vi "Mindsensors PSPNX Config.vi"(10 "Node Data":T1, 11 "NXT":T2) -> ()   [LabVIEW 2010]
uses:
  <vilib>/NXT/Subs/LVHSConnector.ctl
  Datatypes/Node.ctl
  UI Controls/PlugInControls/Pluginbackground.ctl
  <vilib>/Utility/miscctls.llb/LVPointTypeDef.ctl
  <vilib>/NXT/Block Support/HWPage.SensorMode.ctl
  <vilib>/NXT/Block Support/HWPage.SensorType.ctl
  ConvertNodeAddrSensor.vi
panel:
  out "NXT Port":i16
  out "Right Y":dbl
  out "Right X":dbl
  out "Left Y":dbl
  out "Left X":dbl
  in  "Device Address":string
  in  "Device\n Address":u8=2 format="%x"
  in  "Sensor Parameters":string
  out "number":i8
  out "R 3":bool
  out "L 3":bool
  out "R 2":bool
  out "L 1":bool
  out "R 1":bool
  out "L 2":bool
  out "Start":bool
  out "Select":bool
  out "R":bool
  out "U":bool
  out "L":bool
  out "D":bool
  out "[]":bool
  out "O":bool
  out "^":bool
  out "X":bool
  in  "Name":string
  out "Headline":string="Type (auto populated)"
  in  "Instance Specific Data":cluster{"Example Data":dbl}
  in  "Reset":bool
  in  "Save":bool
  in  "Stop":bool
  out "Background":T3=TRUE
  # "<- No controls below this line"
  # "Common controls such as Buttons, Rings, Sliders, Graphs, Decorations, etc can be found in the <labview>\\Targets\\NI\\NXT\\NXT Toolkit\\Schematic Editor\\UI Controls\\Plugin Controls\\ folder. Use these controls when possible to ensure a consistent look and feel with LabVIEW Education Edition."
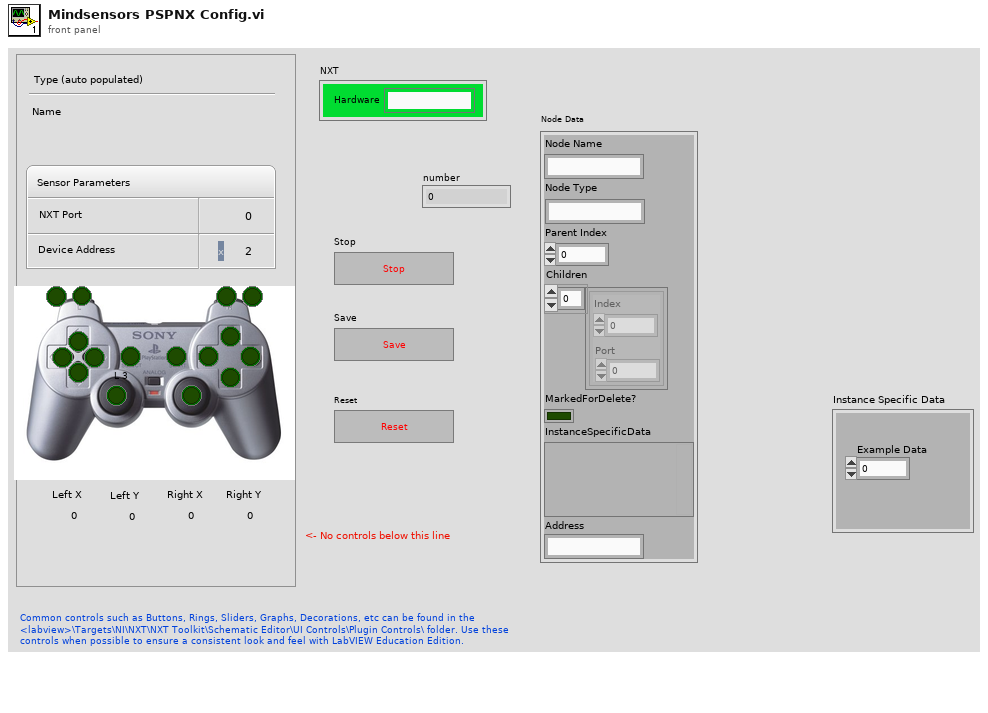
[diagram p1: front panel]
types:
  T1 = typedef "Node.ctl" = cluster{"Node Name":string, "Node Type":string, "Parent Index":i16, "Children":cluster{"Index":u16, "Port":u16}[], "MarkedForDelete?":bool, "InstanceSpecificData":variant, "Address":string}
  T2 = typedef "LVHSConnector.ctl" = cluster{"Hardware":string, "Flattened String":string}
  T3 = typedef "Pluginbackground.ctl" = bool
  T4 = typedef "LVPointTypeDef.ctl" = cluster{"Horizontal":i16, "Vertical":i16}
  T5 = enum8{"Enabled", "Disabled", "Disabled and Grayed Out"}
  T6 = typedef "HWPage.SensorMode.ctl" = u8
  T7 = typedef "HWPage.SensorType.ctl" = u8
  T8 = typedef "NXT_InputPort.ctl" = u8
  T9 = typedef "nxt.ctl" = cluster{"nxtHandle":u32, "fileHandle":u32, "fileIterHandle":u32, "moduleHandle":u32, "modIterHandle":u32, "nxtIterHandle":u32}
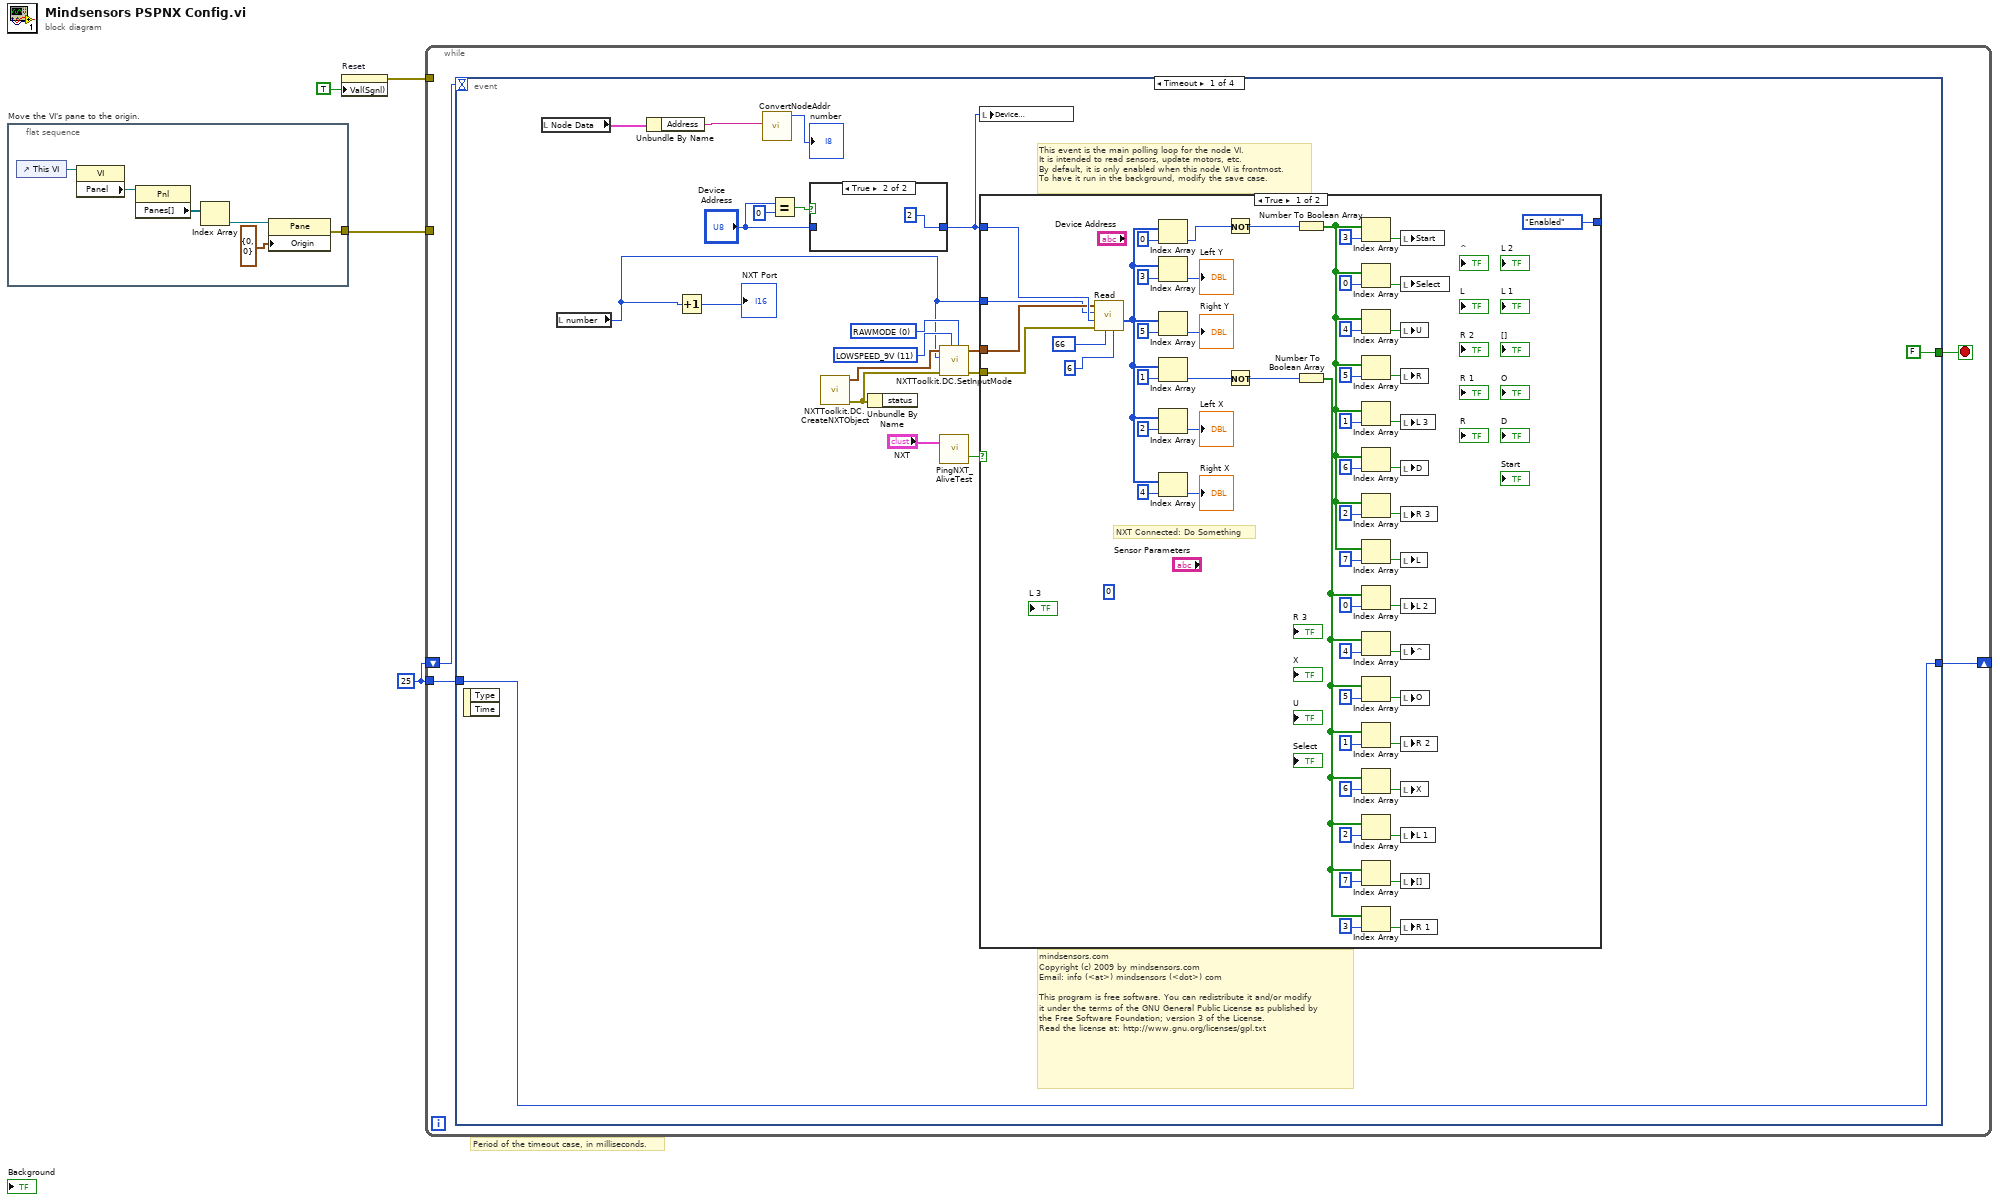
[diagram p0: block diagram]
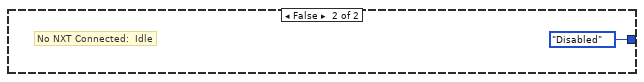
[diagram p3: hidden frame]
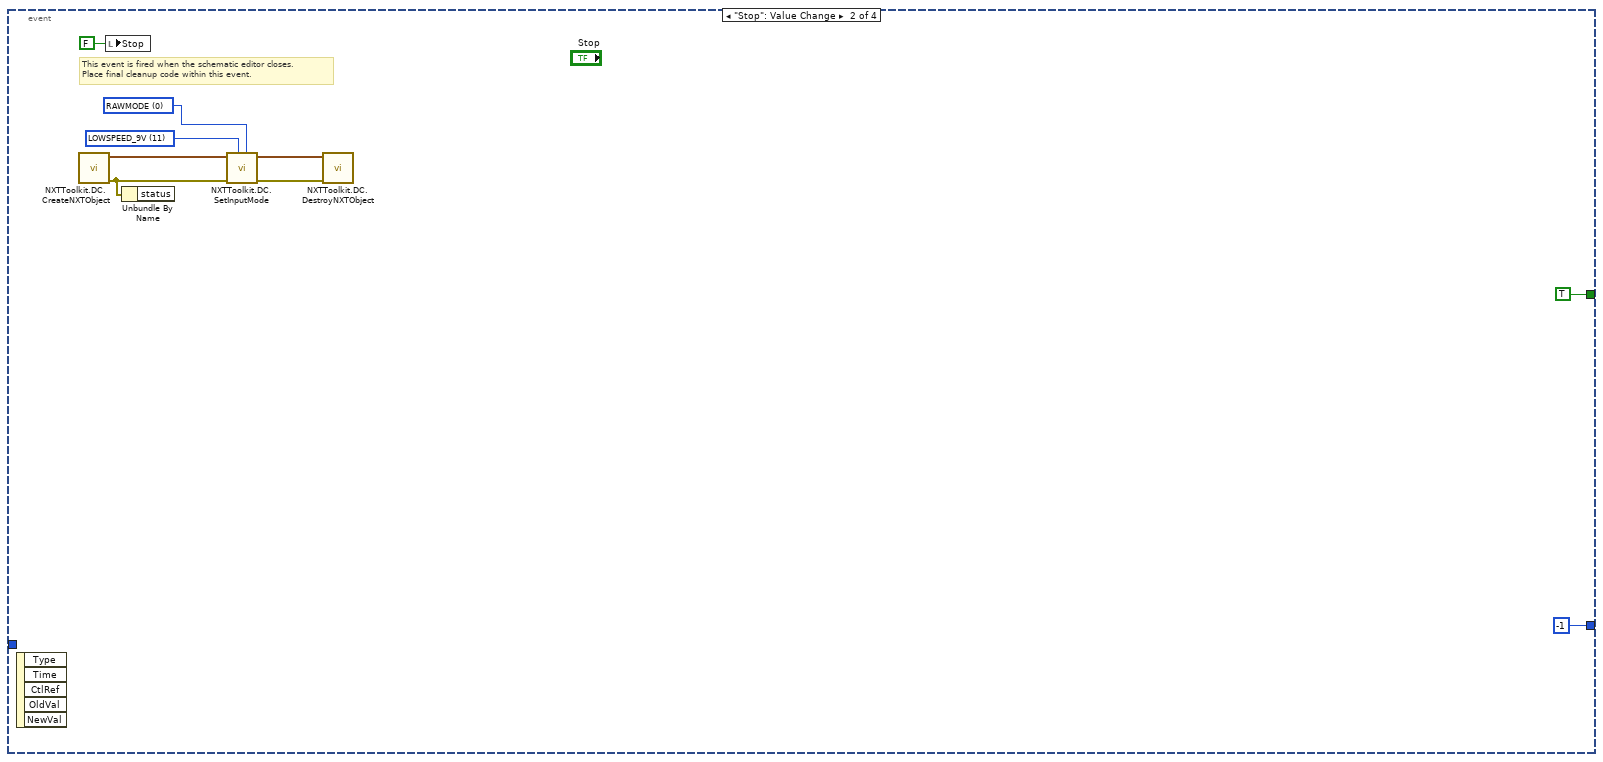
[diagram p4: hidden frame]
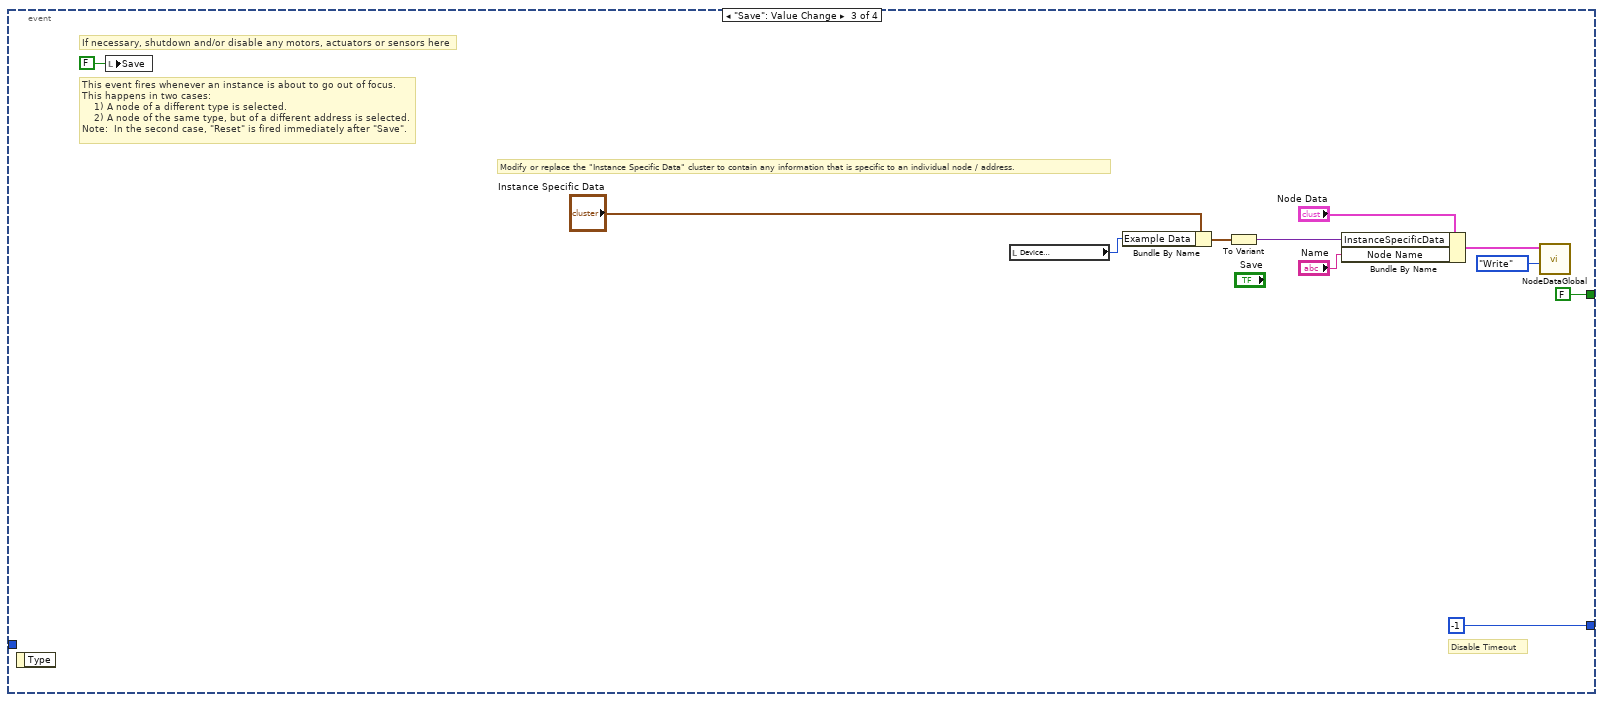
[diagram p5: hidden frame]
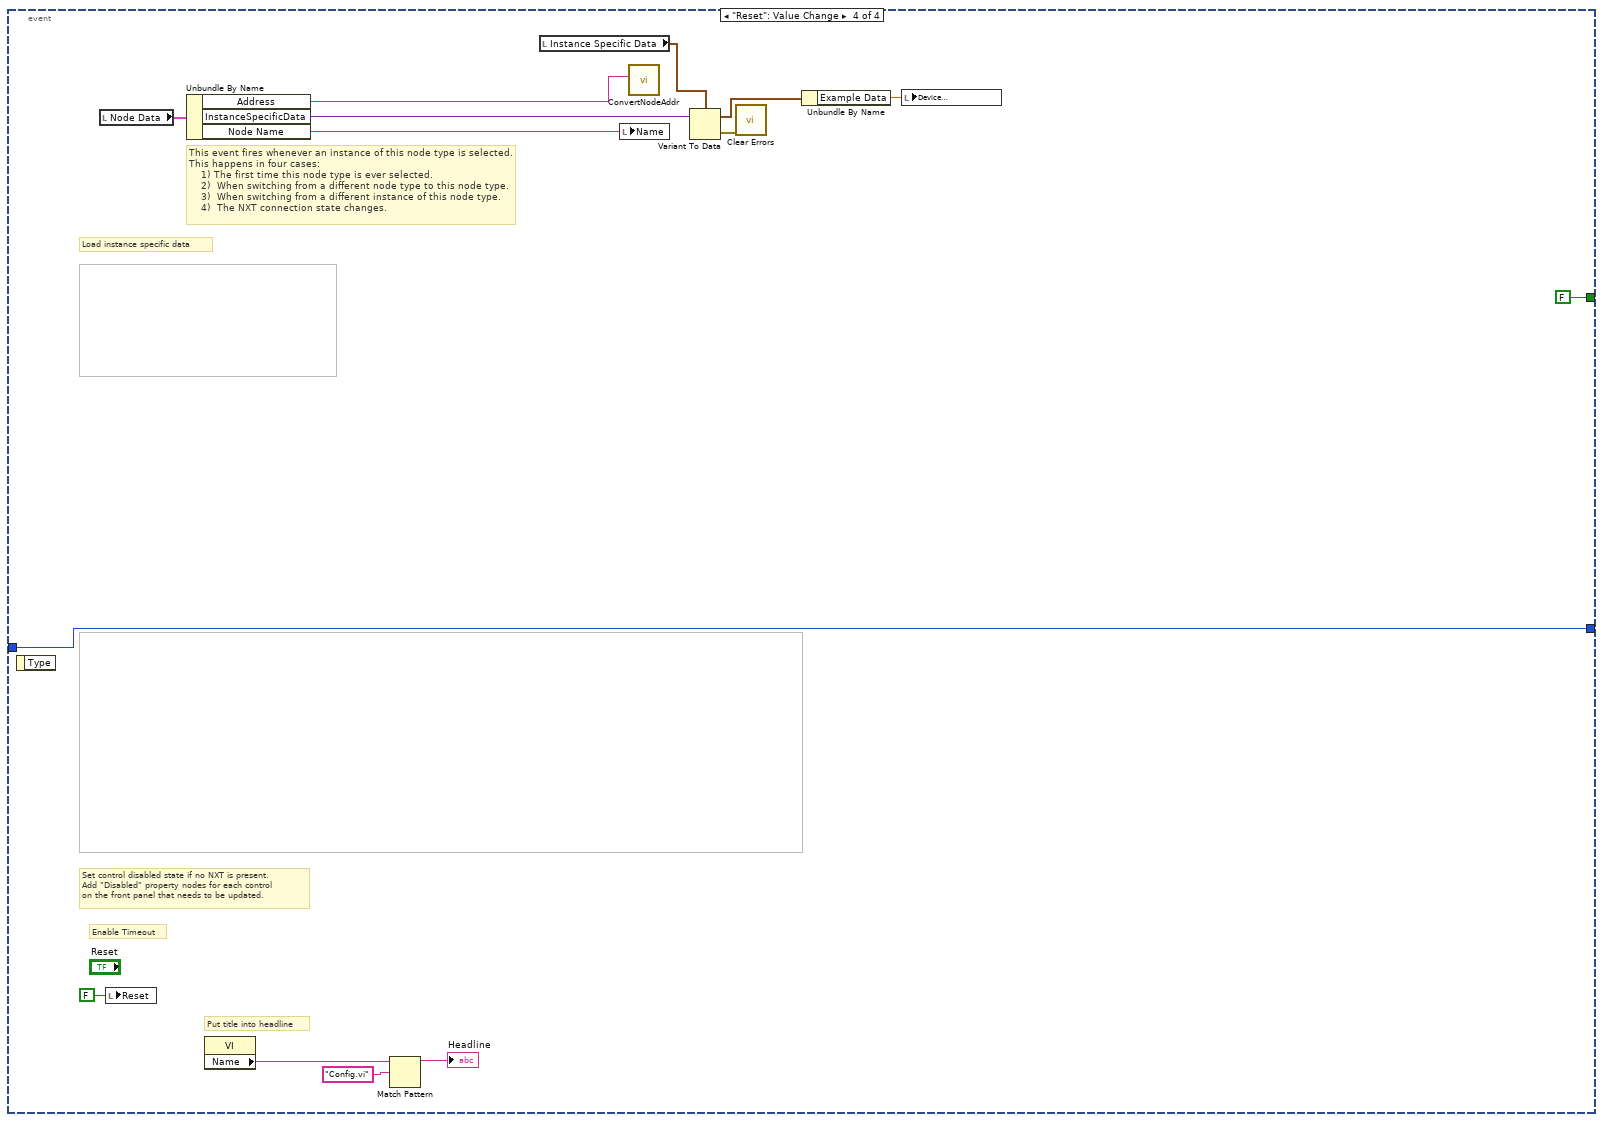
[diagram p6: hidden frame]
diagram:
  w3 = 25
  # "Period of the timeout case, in milliseconds."
  n1 = flat-sequence "Move the VI's pane to the origin." {
    tunnel: [w5] -> w2
    frame #0 {
      n2 = control-ref of="This VI"() -> (w6:refnum<vi>)
      n3 = property class="VI"(reference=w6) -> ("Panel"=w7:refnum<vi>)  [unwired: 1 in, 2 out]
      n4 = property class="Pnl"(reference=w7) -> ("Panes[]"=w8:refnum<vi>[])  [unwired: 1 in, 2 out]
      n5 = Index Array(array=w8) -> (element=w9:refnum<vi>)  [unwired: 1 in]
      n6 = property class="Pane"(reference=w9, "Origin"=T4 {"Horizontal"=0, "Vertical"=0}) -> (error out=w5:errorcluster)  [unwired: 1 in, 1 out]
    }
  }
  n7 = property on="Reset" class="Bool (strict)"("Val(Sgnl)"=TRUE ("Value (Signaling)")) -> (error out=w4:errorcluster)  [unwired: 2 in, 1 out]
  n8 = while {
    tunnel: w4 -> [_]
    shift-right: [w12] -> _
    shift-left: w3 -> [w13]
    tunnel: w3 -> [w11]
    tunnel: w2 -> [_]
    stop <- w14 stop-if-true
    n9 = event shown="[0] Timeout" {
      selector: _ -> [_ _ _ _]
      dyn-events: _ -> [_ _ _ _]
      timeout: w13 -> [_ _ _ _]
      tunnel: [FALSE TRUE FALSE FALSE] -> w14
      tunnel: [w32 -1 -1 w122] -> w12
      tunnel: w11 -> [w32 _ _ w122]
      event Timeout {
        w28 = T6 0 items=["RAWMODE"=0, "BOOLEANMODE"=32, "TRANSITIONCNTMODE"=64, "PERIODCOUNTERMODE"=96, "PCTFULLSCALEMODE"=128, "CELSIUSMODE"=160, "FAHRENHEITMODE"=192, "ANGLESTEPMODE"=224] ("Sensor Mode (RAWMODE)")
        w27 = T7 11 items=["NO_SENSOR", "SWITCH", "TEMPERATURE", "REFLECTION", "ANGLE", "LIGHT_ACTIVE", "LIGHT_INACTIVE", "SOUND_DB", "SOUND_DBA", "CUSTOM", "LOWSPEED", "LOWSPEED_9V", "HIGHSPEED"] ("Sensor Type (NO_SENSOR)")
        # "mindsensors.com\nCopyright (c) 2009 by mindsensors.com\nEmail: info (<at>) mindsensors (<dot>) com\n\nThis program is free software. You can redistribute it and/or modify\nit under the terms of the GNU General Public License as published by\nthe Free Software Foundation; version 3 of the License.\nRead the license at: http://www.gnu.org/licenses/gpl.txt"
        # "This event is the main polling loop for the node VI.\nIt is intended to read sensors, update motors, etc.\nBy default, it is only enabled when this node VI is frontmost.\nTo have it run in the background, modify the save case."
        n10 = event-data() -> ()  [unwired: 1 in, 2 out]
        n11 = local read "Node Data"() -> (w30:T1)
        n12 = local read "number"() -> (w16:i8)
        n13 = Unbundle By Name(w30) -> ("Address"=w18:string)
        n14 = Increment(x=w16) -> (x+1=→"NXT Port":i8)
        n15 = call-poly "ConvertNodeAddr.vi"("Sensor Port"=w18) -> ("NXT Port"=→"number":T8)  [unwired: 6 in, 4 out]
        n16 = Equal?(x="Device\n Address", y=u8 0) -> (x = y?=w21:bool)
        n17 = case shown="True" w21 {
          tunnel: [w34 u8 2 ("Device Addr 2")] -> w19
          tunnel: "Device\n Address" -> [w34 _]
          frame False {
          }
          frame True {
          }
        }
        n18 = call <vilib>:"NXTToolkit.DC.CreateNXTObject.vi"() -> ("error out"=w25:errorcluster, "NXTObject"=w26:T9)  [unwired: 9 in, 1 out]
        n19 = Unbundle By Name(w25) -> ()  [unwired: 1 out]
        n20 = call <vilib>:"NXTToolkit.DC.SetInputMode.vi"("Sensor Mode (RAWMODE)"=w28, "Sensor Type (NO_SENSOR)"=w27, "error in (no error)"=w25, "Input Port (Port 1)"=w16, "NXTObject"=w26) -> ("error out"=w23:errorcluster, "NXTObject dup"=w24:T9)  [unwired: 4 in, 1 out]
        n21 = call <vilib>:"PingNXT_AliveTest.vi"("NXT"="NXT") -> ("connected?"=w29:bool)  [unwired: 1 in, 1 out]
        n22 = local write "Device\n Address"(w19) -> ()
        n23 = case shown="True" w29 {
          tunnel: [T5."Enabled" ("Disabled") T5."Disabled" ("Disabled")] -> _
          tunnel: w16 -> [w36 _]
          tunnel: w19 -> [w90 _]
          tunnel: w24 -> [w38 _]
          tunnel: w23 -> [w37 _]
          frame True {
            (unwired) 0 ("index")
            # "NXT Connected: Do Something"
            n24 = call <vilib>:"Read.vi"("bytes to read"=u8 6, "Reg Address"=u8 66, "error in (no error)"=w37, "Device Address"=w90, "Input Port in"=w36, "NXTObject"=w38) -> ("data Buffer"=w79:u8[])  [unwired: 5 out]
            n25 = Index Array(array=w79, index=0) -> (element=w81:u8)
            n26 = Index Array(array=w79, index=3) -> (element=→"Left Y":u8)
            n27 = Index Array(array=w79, index=5) -> (element=→"Right Y":u8)
            n28 = Index Array(array=w79, index=1) -> (element=w80:u8)
            n29 = Index Array(array=w79, index=2) -> (element=→"Left X":u8)
            n30 = Index Array(array=w79, index=4) -> (element=→"Right X":u8)
            n31 = Not(x=w81) -> (.not. x?=w74:u8)
            n32 = Not(x=w80) -> (.not. x?=w73:u8)
            n33 = Number To Boolean Array(number=w74) -> (Boolean array=w56:bool[])
            n34 = Number To Boolean Array(number=w73) -> (Boolean array=w39:bool[])
            n35 = Index Array(array=w56, index=3) -> (element=w62:bool)
            n36 = Index Array(array=w56, index=0) -> (element=w63:bool)
            n37 = Index Array(array=w56, index=4) -> (element=w60:bool)
            n38 = Index Array(array=w56, index=5) -> (element=w61:bool)
            n39 = Index Array(array=w56, index=1) -> (element=w70:bool)
            n40 = Index Array(array=w56, index=6) -> (element=w59:bool)
            n41 = Index Array(array=w56, index=2) -> (element=w69:bool)
            n42 = Index Array(array=w56, index=7) -> (element=w57:bool)
            n43 = Index Array(array=w39, index=0) -> (element=w47:bool)
            n44 = Index Array(array=w39, index=4) -> (element=w42:bool)
            n45 = Index Array(array=w39, index=5) -> (element=w43:bool)
            n46 = Index Array(array=w39, index=1) -> (element=w46:bool)
            n47 = Index Array(array=w39, index=6) -> (element=w41:bool)
            n48 = Index Array(array=w39, index=2) -> (element=w45:bool)
            n49 = Index Array(array=w39, index=7) -> (element=w40:bool)
            n50 = Index Array(array=w39, index=3) -> (element=w44:bool)
            n51 = local write "Start"(w62) -> ()
            n52 = local write "Select"(w63) -> ()
            n53 = local write "U"(w60) -> ()
            n54 = local write "R"(w61) -> ()
            n55 = local write "L 3"(w70) -> ()
            n56 = local write "D"(w59) -> ()
            n57 = local write "R 3"(w69) -> ()
            n58 = local write "L"(w57) -> ()
            n59 = local write "L 2"(w47) -> ()
            n60 = local write "^"(w42) -> ()
            n61 = local write "O"(w43) -> ()
            n62 = local write "R 2"(w46) -> ()
            n63 = local write "X"(w41) -> ()
            n64 = local write "L 1"(w45) -> ()
            n65 = local write "[]"(w40) -> ()
            n66 = local write "R 1"(w44) -> ()
          }
          frame False {
            # "No NXT Connected:  Idle"
          }
        }
      }
      event "Stop": Value Change {
        w98 = T6 0 items=["RAWMODE"=0, "BOOLEANMODE"=32, "TRANSITIONCNTMODE"=64, "PERIODCOUNTERMODE"=96, "PCTFULLSCALEMODE"=128, "CELSIUSMODE"=160, "FAHRENHEITMODE"=192, "ANGLESTEPMODE"=224] ("Sensor Mode (RAWMODE)")
        w97 = T7 11 items=["NO_SENSOR", "SWITCH", "TEMPERATURE", "REFLECTION", "ANGLE", "LIGHT_ACTIVE", "LIGHT_INACTIVE", "SOUND_DB", "SOUND_DBA", "CUSTOM", "LOWSPEED", "LOWSPEED_9V", "HIGHSPEED"] ("Sensor Type (NO_SENSOR)")
        # "This event is fired when the schematic editor closes.\nPlace final cleanup code within this event."
        n67 = event-data() -> ()  [unwired: 1 in, 5 out]
        n68 = call <vilib>:"NXTToolkit.DC.CreateNXTObject.vi"() -> ("error out"=w95:errorcluster, "NXTObject"=w96:T9)  [unwired: 9 in, 1 out]
        n69 = local write "Stop"(FALSE ("stop")) -> ()
        n70 = Unbundle By Name(w95) -> ()  [unwired: 1 out]
        n71 = call <vilib>:"NXTToolkit.DC.SetInputMode.vi"("Sensor Mode (RAWMODE)"=w98, "Sensor Type (NO_SENSOR)"=w97, "error in (no error)"=w95, "NXTObject"=w96) -> ("error out"=w93:errorcluster, "NXTObject dup"=w94:T9)  [unwired: 5 in, 1 out]
        n72 = call <vilib>:"NXTToolkit.DC.DestroyNXTObject.vi"("error in (no error)"=w93, "NXTObject"=w94) -> ()  [unwired: 9 in, 1 out]
      }
      event "Save": Value Change {
        # "If necessary, shutdown and/or disable any motors, actuators or sensors here"
        # "Modify or replace the \"Instance Specific Data\" cluster to contain any information that is specific to an individual node / address."
        # "Disable Timeout"
        # "This event fires whenever an instance is about to go out of focus.\nThis happens in two cases:\n    1) A node of a different type is selected.\n    2) A node of the same type, but of a different address is selected.\nNote:  In the second case, \"Reset\" is fired immediately after \"Save\"."
        n73 = event-data() -> ()  [unwired: 1 in, 1 out]
        n74 = local write "Save"(FALSE ("stop")) -> ()
        n75 = local read "Device\n Address"() -> (w102:u8)
        n76 = Bundle By Name(cluster="Instance Specific Data", "Example Data"=w102) -> (w103:cluster{"Example Data":dbl})
        n77 = To Variant(anything=w103) -> (Variant=w110:variant)
        n78 = Bundle By Name(cluster="Node Data", "InstanceSpecificData"=w110, "Node Name"="Name") -> (w109:T1)
        n79 = call "NodeDataGlobal.vi"("Action"=enum16{"Read", "Write"}."Write", "Node Data In"=w109) -> ()  [unwired: 8 in, 2 out]
      }
      event "Reset": Value Change {
        # "Set control disabled state if no NXT is present.\nAdd \"Disabled\" property nodes for each control\non the front panel that needs to be updated."
        # "Load instance specific data"
        # "Enable Timeout"
        # "This event fires whenever an instance of this node type is selected.\nThis happens in four cases:\n    1) The first time this node type is ever selected.\n    2)  When switching from a different node type to this node type.\n    3)  When switching from a different instance of this node type. \n    4)  The NXT connection state changes."
        # "Put title into headline"
        n80 = event-data() -> ()  [unwired: 1 in, 1 out]
        n81 = local read "Node Data"() -> (w123:T1)
        n82 = local write "Reset"(FALSE ("Reset")) -> ()
        n83 = Unbundle By Name(w123) -> ("Address"=w114:string, "InstanceSpecificData"=w124:variant, "Node Name"=w116:string)
        n84 = property class="VI"() -> ("Name"=w118:string)  [unwired: 2 in, 2 out]
        n85 = Match Pattern(string=w118, regular expression="Config.vi") -> (before substring=→"Headline":string)  [unwired: 1 in, 3 out]
        n86 = local read "Instance Specific Data"() -> (w121:cluster{"Example Data":dbl})
        n87 = local write "Name"(w116) -> ()
        n88 = call-poly "ConvertNodeAddr.vi"("Sensor Port"=w114) -> ()  [unwired: 6 in, 5 out]
        n89 = Variant To Data(Variant=w124, type=w121) -> (error out=w120:errorcluster, data=w115:cluster{"Example Data":dbl})  [unwired: 1 in]
        n90 = call <vilib>:"Clear Errors.vi"("error in (no error)"=w120) -> ()  [unwired: 6 in, 1 out]
        n91 = Unbundle By Name(w115) -> ("Example Data"=w113:dbl)
        n92 = local write "Device\n Address"(w113) -> ()
      }
    }
  }
